vi "Exercise1.15-Shift Register  Accumulator.vi"() -> ()   [LabVIEW 2013]
panel:
  out "Sum":i32
  in  "N":i32
  in  "N":i32
  out "Sum":i32
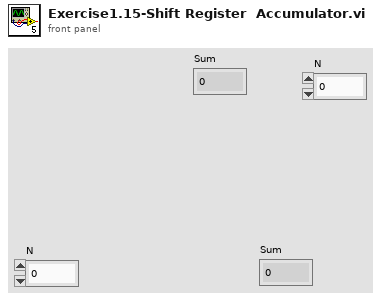
[diagram p1: front panel]
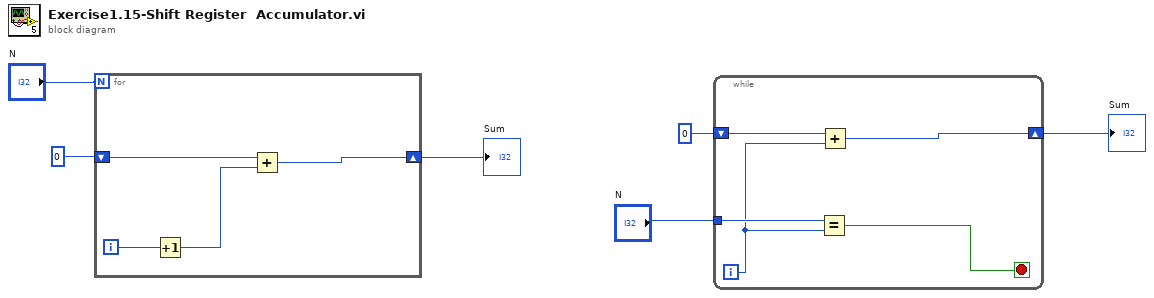
[diagram p0: block diagram]
diagram:
  n1 = for {
    N: "N" -> [_]
    shift-right: [w7] -> w1
    shift-left: 0 -> [w8]
    i -> [w10]
    n2 = Increment(x=w10) -> (x+1=w9:i32)
    n3 = Add(x=w8, y=w9) -> (x+y=w7:i32)
  }
  "Sum" <- w1
  n4 = while {
    shift-right: [w14] -> w5
    shift-left: 0 -> [w15]
    tunnel: "N" -> [w12]
    i -> [w11]
    stop <- w13 stop-if-true
    n5 = Equal?(x=w12, y=w11) -> (x = y?=w13:bool)
    n6 = Add(x=w15, y=w11) -> (x+y=w14:i32)
  }
  "Sum" <- w5
